vi "Norm Sub Vector Calcul.vi"(8 "u21":dbl format="%#_13g", 9 "u12":dbl format="%#_13g", 10 "m2":dbl format="%#_13g", 11 "m1":dbl format="%#_13g") -> (2 "v21":dbl, 3 "v12":dbl)   [LabVIEW 2021, in "Game Board.lvclass"]
doc: "MIT Licence\nCopyright (c) 2024 David Grollier"
uses:
  Game Board.lvclass
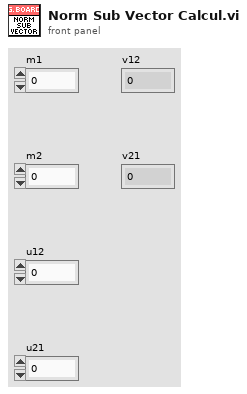
[diagram p1: front panel]
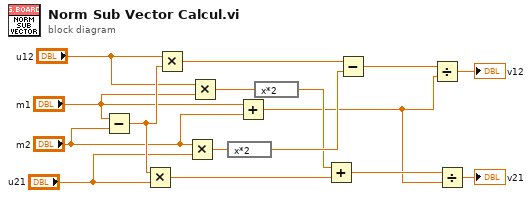
[diagram p0: block diagram]
diagram:
  n1 = Subtract(x="m1", y="m2") -> (x-y=w16:dbl)
  n2 = Multiply(x=w16, y="u21") -> (x*y=w10:dbl)
  n3 = Multiply(x="u12", y=w16) -> (x*y=w15:dbl)
  n4 = Multiply(x="m2", y="u21") -> (x*y=w14:dbl)
  n5 = Multiply(x="u12", y="m1") -> (x*y=w8:dbl)
  n6 = expression code="x*2"(w14) -> (w13:dbl)
  n7 = Add(x="m1", y="m2") -> (x+y=w3:dbl)
  n8 = expression code="x*2"(w8) -> (w9:dbl)
  n9 = Add(x=w9, y=w10) -> (x+y=w4:dbl)
  n10 = Subtract(x=w15, y=w13) -> (x-y=w5:dbl)
  n11 = Divide(x=w5, y=w3) -> (x/y=→"v12":dbl)
  n12 = Divide(x=w4, y=w3) -> (x/y=→"v21":dbl)
